vi "IO_OpenDevice.vi"(4 "error in":errorcluster caption="错误输入", 7 "ComNum":i32=1) -> (0 "error out":errorcluster caption="错误输出", 3 "hDevice":u32 format="%x")   [LabVIEW 2013]
uses:
  FY2400P.dll
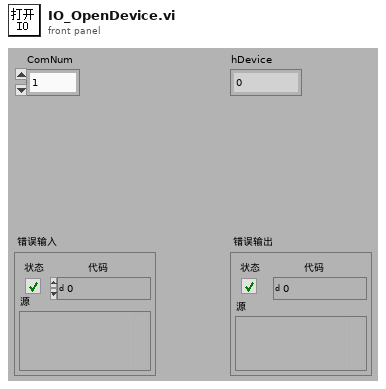
[diagram p1: front panel]
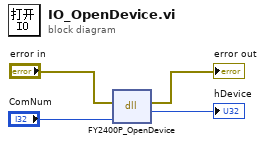
[diagram p0: block diagram]
diagram:
  n1 = dll-call lib="PTH1\\abs E桌面休眠电流方案休眠电流源码20181130\nInstrumentIOFY2400P.dll" fn="FY2400P_OpenDevice"(error in="error in", "Comnum"="ComNum") -> (error out=→"error out":errorcluster, "返回类型"=→"hDevice":u32)  [unwired: 3 in, 1 out]
